vi "CMD_RSM_SE4500_GENERIC_Command.vi"(0 "Input_Data":string[](array[string]), 5 "Error In":errorcluster) -> (12 "Validate CheckSum":bool, 13 "Command":u8[](array[numeric])=[4, 228, 4, 128, 0, 0, 0, 0, 0, 0, 0, 0, 0, 0] format="%x", 14 "Response":bool, 15 "Ack":bool, 16 "Command":bool, 17 "Add CheckSum":bool, 18 "Status":bool, 19 "Error Out":errorcluster)   [LabVIEW 2014]
panel:
  # "Flags"
  # "RSM_SE4500_Generic Command:"
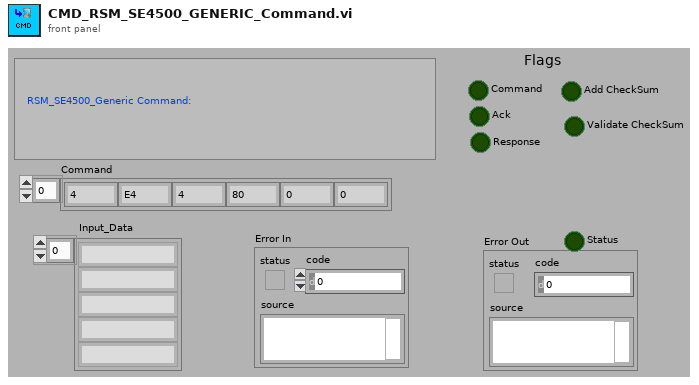
[diagram p1: front panel]
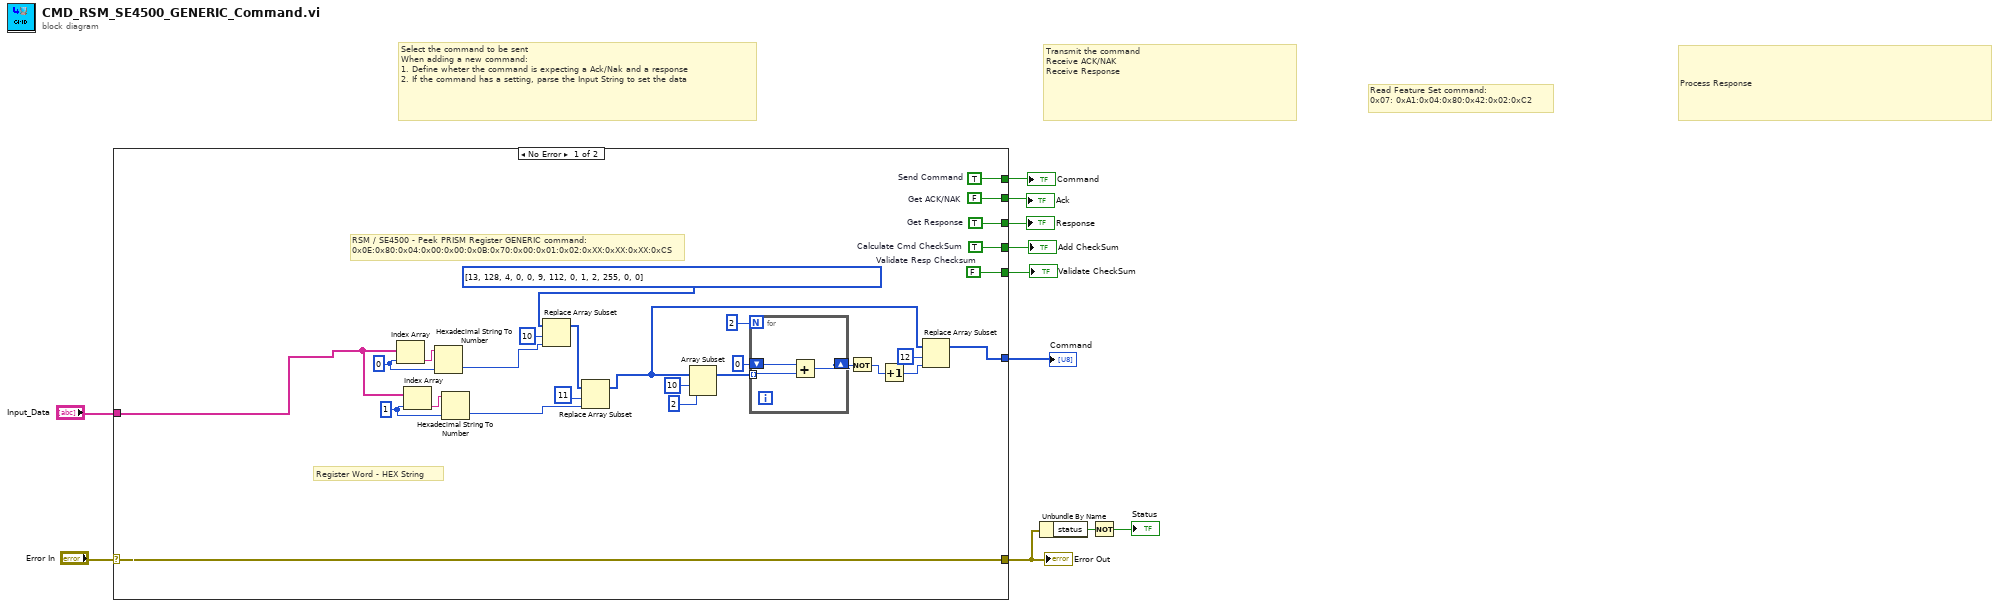
[diagram p0: block diagram]
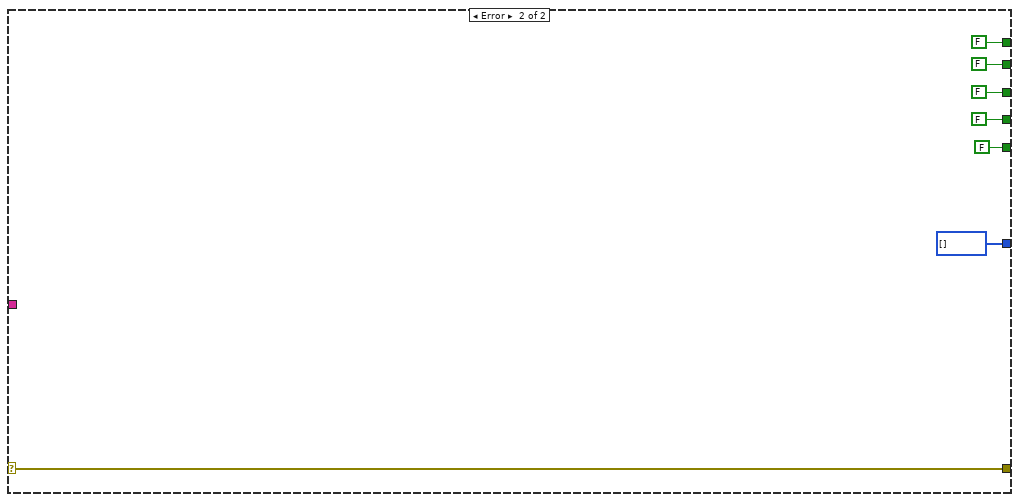
[diagram p2: hidden frame]
diagram:
  # "Read Feature Set command:\n0x07: 0xA1:0x04:0x80:0x42:0x02:0xC2"
  # "Process Response"
  # "Transmit the command\nReceive ACK/NAK\nReceive Response"
  # "Select the command to be sent\nWhen adding a new command:\n1. Define wheter the command is expecting a Ack/Nak and a response\n2. If the command has a setting, parse the Input String to set the data"
  n1 = case shown="No Error" "Error In" {
    selector: "Error In" -> [w35 w44]
    tunnel: [w39 FALSE ("Send Command")] -> w10
    tunnel: [w38 FALSE ("Get ACK/NAK")] -> w9
    tunnel: [w37 FALSE ("Get Response")] -> w8
    tunnel: [w36 FALSE ("Add CheckSum")] -> w7
    tunnel: [w13 u8[] []] -> w6
    tunnel: [w35 w44] -> w4
    tunnel: "Input_Data" -> [w12 _]
    tunnel: [w34 FALSE ("Validate Resp Checksum")] -> w1
    frame No Error {
      w15 = 1 ("index")
      w19 = 0 ("index")
      w34 = FALSE  # Validate Resp Checksum
      w36 = TRUE  # Calculate Cmd CheckSum
      w37 = TRUE  # Get Response
      w39 = TRUE  # Send Command
      w38 = FALSE  # Get ACK/NAK
      # "Register Word - HEX String"
      # "RSM / SE4500 - Peek PRISM Register GENERIC command:\n0x0E:0x80:0x04:0x00:0x00:0x0B:0x70:0x00:0x01:0x02:0xXX:0xXX:0xXX:0xCS"
      n2 = Index Array(array=w12, index=w19) -> (element=w21:string)
      n3 = Index Array(array=w12, index=w15) -> (element=w16:string)
      n4 = Hexadecimal String To Number(string=w21, default (0uL)=w19) -> (number=w17:i32)  [unwired: 1 in, 1 out]
      n5 = Hexadecimal String To Number(string=w16, default (0uL)=w15) -> (number=w14:i32)  [unwired: 1 in, 1 out]
      n6 = Replace Array Subset(array=u8[] [13, 128, 4, 0, 0, 9, 112, 0, 1, 2, 255, 0, 0], new element=w17, index=10) -> (w22:u8[])
      n7 = Replace Array Subset(array=w22, new element=w14, index=11) -> (w20:u8[])
      n8 = Array Subset(array=w20, index=10, length=2) -> (w25:u8[])
      n9 = for {
        N: 2 -> [_]
        tunnel: w25 -> [w42] mode=indexing
        shift-right: [w40] -> w31
        shift-left: u16 0 -> [w41]
        n10 = Add(x=w41, y=w42) -> (x+y=w40:u16)
      }
      n11 = Not(x=w31) -> (.not. x?=w30:u16)
      n12 = Increment(x=w30) -> (x+1=w29:u16)
      n13 = Replace Array Subset(array=w20, new element=w29, index=12) -> (w13:u8[])
    }
    frame Error {
    }
  }
  "Error Out" <- w4
  "Command" <- w10
  "Ack" <- w9
  "Response" <- w8
  "Add CheckSum" <- w7
  "Command" <- w6
  "Validate CheckSum" <- w1
  n14 = Unbundle By Name(w4) -> ("status"=w3:bool)
  n15 = Not(x=w3) -> (.not. x?=→"Status":bool)
